vi "Trim Sensitivity Characterization Vbias Gain.vi"(0 "TSM context":T1) -> (15 "error out":errorcluster)   [LabVIEW 2020]
uses:
  <vilib>/NI_TestStand_SemiconductorModule/NI_TestStand_Semiconductor_Module.lvlibp/PinMap/General/SemiconductorModuleContext.ctl
  <vilib>/Analysis/1siggen.llb/Ramp Pattern.vi
  <vilib>/Analysis/1siggen.llb/Ramp Pattern by Delta.vi
  <vilib>/Utility/error.llb/Error Cluster From Error Code.vi
  <vilib>/NI_TestStand_SemiconductorModule/NI_TestStand_Semiconductor_Module.lvlibp
panel:
  out "Gain Sweep":dbl[][](array[numeric])
  out "Vbias Sweep":dbl[][](array[numeric])
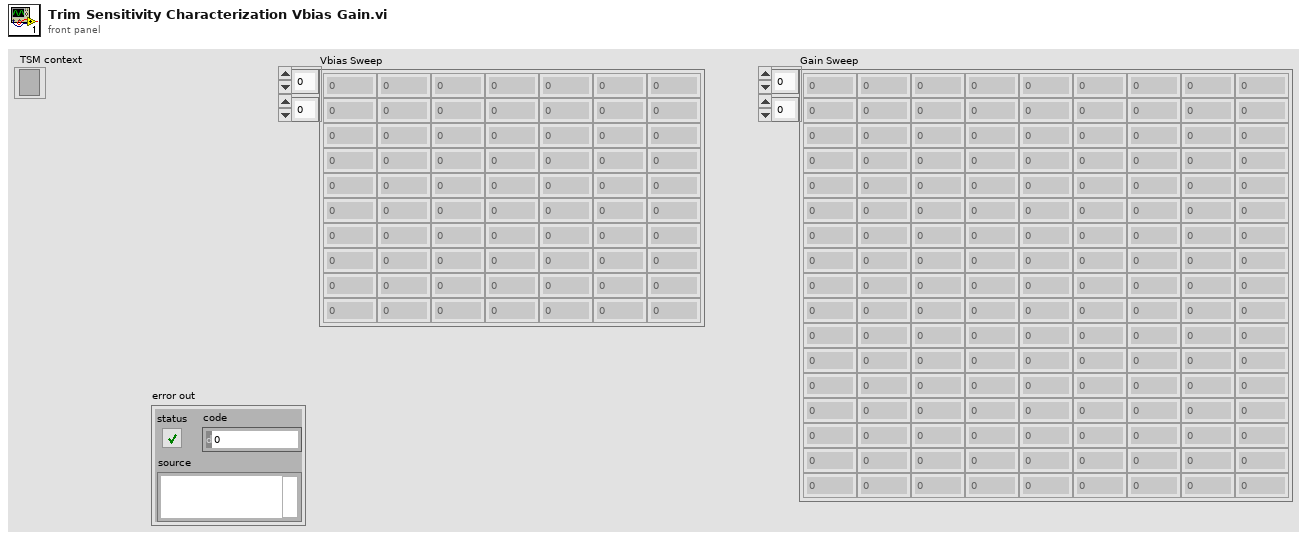
[diagram p1: front panel]
types:
  T1 = typedef "NI_TestStand_Semiconductor_Module.lvlibp/SemiconductorModuleContext.ctl" = refnum<k7>
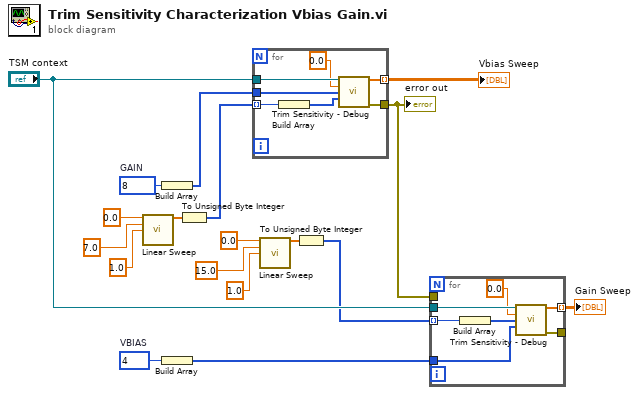
[diagram p0: block diagram]
diagram:
  w8 = u8 4  # VBIAS
  w17 = u8 8  # GAIN
  n1 = call "Linear Sweep.vi"("Start"=0.0, "End"=7.0, "Delta"=1.0) -> ("Ramp Pattern"=w12:dbl[])  [unwired: 11 in, 1 out]
  n2 = Build Array(w17) -> (w16:u8[])
  n3 = Build Array(w8) -> (w7:u8[])
  n4 = To Unsigned Byte Integer(number=w12) -> (unsigned 8bit integer=w11:u8[])
  n5 = for {
    tunnel: [w25] -> w10
    tunnel: "TSM context" -> [w24]
    tunnel: [w23] -> w18 mode=indexing
    tunnel: w16 -> [w22]
    tunnel: w11 -> [w21] mode=indexing
    n6 = Build Array(w21) -> (w20:u8[])
    n7 = call "Trim Sensitivity - Debug.vi"("TSM context"=w24, "Target Sensitivity (dBV)"=0.0, "Gain"=w22, "Vbias"=w20) -> ("Trimmed dB V"=w23:dbl[], "error out"=w25:errorcluster)  [unwired: 10 in]
  }
  "error out" <- w10
  "Vbias Sweep" <- w18
  n8 = call "Linear Sweep.vi"("Start"=0.0, "End"=15.0, "Delta"=1.0) -> ("Ramp Pattern"=w6:dbl[])  [unwired: 11 in, 1 out]
  n9 = To Unsigned Byte Integer(number=w6) -> (unsigned 8bit integer=w2:u8[])
  n10 = for {
    tunnel: [w32] -> _
    tunnel: "TSM context" -> [w31]
    tunnel: [w30] -> w1 mode=indexing
    tunnel: w2 -> [w29] mode=indexing
    tunnel: w10 -> [_]
    tunnel: w7 -> [w27]
    n11 = Build Array(w29) -> (w26:u8[])
    n12 = call "Trim Sensitivity - Debug.vi"("TSM context"=w31, "Target Sensitivity (dBV)"=0.0, "Gain"=w26, "Vbias"=w27) -> ("Trimmed dB V"=w30:dbl[], "error out"=w32:errorcluster)  [unwired: 10 in]
  }
  "Gain Sweep" <- w1
